vi "BRAM Address Select.vi"(5 "Write Address":u16, 7 "Read Address":u16, 9 "Read/Write?":T1=enum."Read from Bank") -> (6 "BRAM Address":u16, 10 "Write?":bool)   [LabVIEW 2011]
uses:
  <userlib>/FPGA Library/Code Development/Signal Processing/FFT/Real Sequence from Complex FFT/BRAM State.ctl
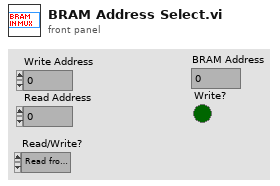
[diagram p1: front panel]
types:
  T1 = typedef "BRAM State.ctl" = enum8{"Write to Bank", "Read from Bank"}
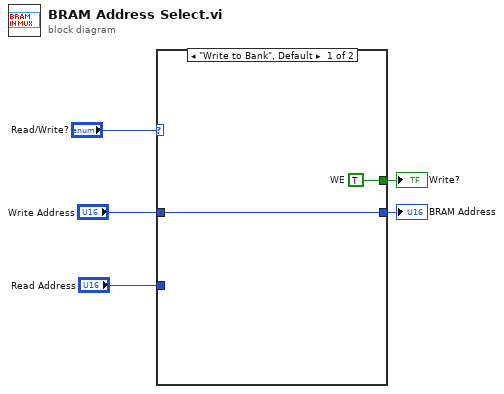
[diagram p0: block diagram]
diagram:
  n1 = case shown="\"Write to Bank\", Default" "Read/Write?" {
    tunnel: [w7 _] -> w2
    tunnel: "Read Address" -> [_ w8]
    tunnel: [w6 w8] -> w3
    tunnel: "Write Address" -> [w6 _]
    frame "Write to Bank", Default {
      w7 = TRUE  # WE
    }
    frame "Read from Bank" {
    }
  }
  "BRAM Address" <- w3
  "Write?" <- w2
